vi "Parse Markdown Note Elements.vi"(8 "Error in":errorcluster caption="Error in (no error)", 11 "Lines":string[](array[string])) -> (0 "Error out":errorcluster, 2 "Array":T1[](array[typedef]), 3 "Lines (dup)":string[](array[string]))   [LabVIEW 2017]
uses:
  _Typedef/DocNote.ctl
  csmdoc.lvlib
  Communicable State Machine.lvlib
  _Shared/CSM Shared.lvlib
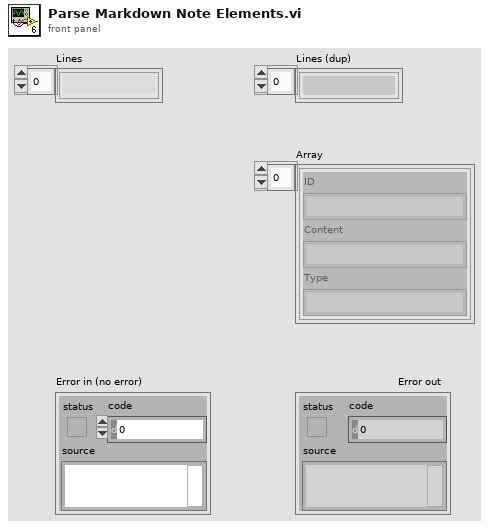
[diagram p1: front panel]
types:
  T1 = typedef "csmdoc.lvlib/DocNote.ctl" = cluster{"ID":string, "Content":string, "Type":string}
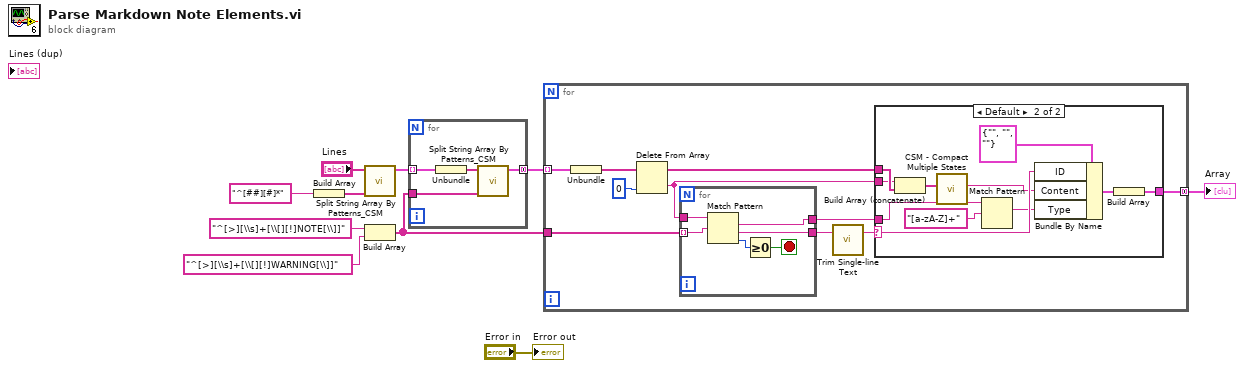
[diagram p0: block diagram]
diagram:
  n1 = Build Array("^[##][#]*" ("delimited string")) -> (w3:string[])
  n2 = call "Split String Array By Patterns_CSM.vi"("Patterns"=w3, "Text Array"="Lines") -> ("Array"=w4:cluster{"filtered array":string[]}[])  [unwired: 9 in]
  n3 = Build Array("^[>][\\s]+[\\[][!]NOTE[\\]]" ("delimited string"), "^[>][\\s]+[\\[][!]WARNING[\\]]" ("delimited string")) -> (w9:string[])
  n4 = for {
    tunnel: w4 -> [w14] mode=indexing
    tunnel: [w12] -> w5 mode=concatenating
    tunnel: w9 -> [w11]
    n5 = Unbundle(w14) -> ("filtered array"=w13:string[])
    n6 = call "Split String Array By Patterns_CSM.vi"("Patterns"=w11, "Text Array"=w13) -> ("Array"=w12:cluster{"filtered array":string[]}[])  [unwired: 9 in]
  }
  n7 = for {
    tunnel: w5 -> [w24] mode=indexing
    tunnel: [w17] -> w10 mode=concatenating
    tunnel: w9 -> [w16]
    n8 = Unbundle(w24) -> ("filtered array"=w23:string[])
    n9 = Delete From Array(array=w23, index=0) -> (deleted portion=w19:string, array with subset deleted=w20:string[])  [unwired: 1 in]
    n10 = for {
      tunnel: w19 -> [w29]
      tunnel: [w30] -> w21
      tunnel: w16 -> [w28] mode=indexing
      tunnel: [w25] -> w15
      stop <- w26 stop-if-true
      n11 = Match Pattern(string=w29, regular expression=w28) -> (match substring=w25:string, after substring=w30:string, offset past match=w27:i32)  [unwired: 1 in, 1 out]
      n12 = Greater Or Equal To 0?(x=w27) -> (x >= 0?=w26:bool)
    }
    n13 = call "Trim Single-line Text.vi"("single-line text"=w21) -> ("trimed text"=w18:string)  [unwired: 2 in]
    n14 = case shown="Default" w18 {
      selector: w18 -> [_ w37]
      tunnel: w20 -> [_ w41]
      tunnel: w19 -> [_ w39]
      tunnel: [_ w34] -> w17
      tunnel: w15 -> [_ w32]
      frame "" {
      }
      frame Default {
        n15 = Build Array (concatenate)(w39, w41) -> (w40:string[])
        n16 = call "CSM - Compact Multiple States.vi"("Multiple States"=w40) -> ("States"=w36:string)  [unwired: 9 in]
        n17 = Match Pattern(string=w32, regular expression="[a-zA-Z]+") -> (match substring=w31:string)  [unwired: 1 in, 3 out]
        n18 = Bundle By Name(cluster=T1 {"ID"="", "Content"="", "Type"=""} ("Cluster"), "ID"=w37, "Content"=w36, "Type"=w31) -> (w35:T1)
        n19 = Build Array(w35) -> (w34:T1[])
      }
    }
  }
  "Array" <- w10
  "Error out" <- "Error in"
